vi "MSScript_Format_UpdAuxArbPulses.vi"(9 "ValueArray":string[](array[string]), 10 "TagArray":string[](array[string]), 11 "MSScript.lvclass":refnum<class "MSScript.lvclass">) -> (0 "ValueErrorArray":bool[](array[boolean]), 1 "TagErrorArray":bool[](array[boolean]), 2 "ParamErrorArray":bool[](array[boolean]), 3 "Data":variant, 4 "#ofParamError":bool)   [LabVIEW 2018, in "MSScript.lvclass"]
uses:
  MSScript.lvclass
  Ctl/MSEditorParam updAuxArbPulses.ctl
  MSScript_Transform_EXTArray.vi
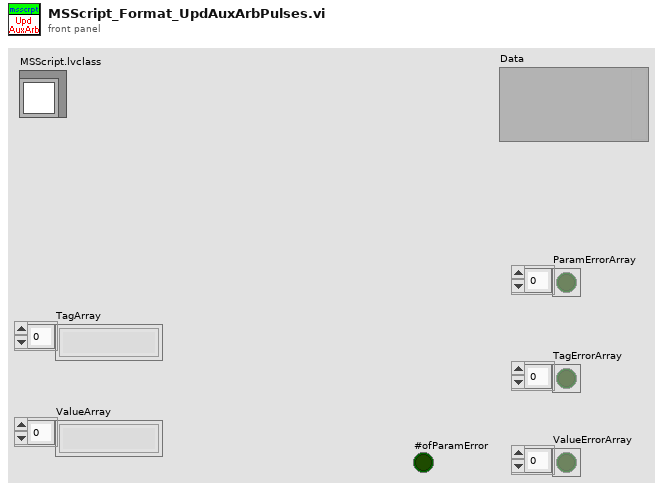
[diagram p1: front panel]
types:
  T1 = typedef "MSEditorParam updAuxArbPulses.ctl" = cluster{"cycleIni":ext[], "cycleEnd":ext[], "pulseInt":ext[]}
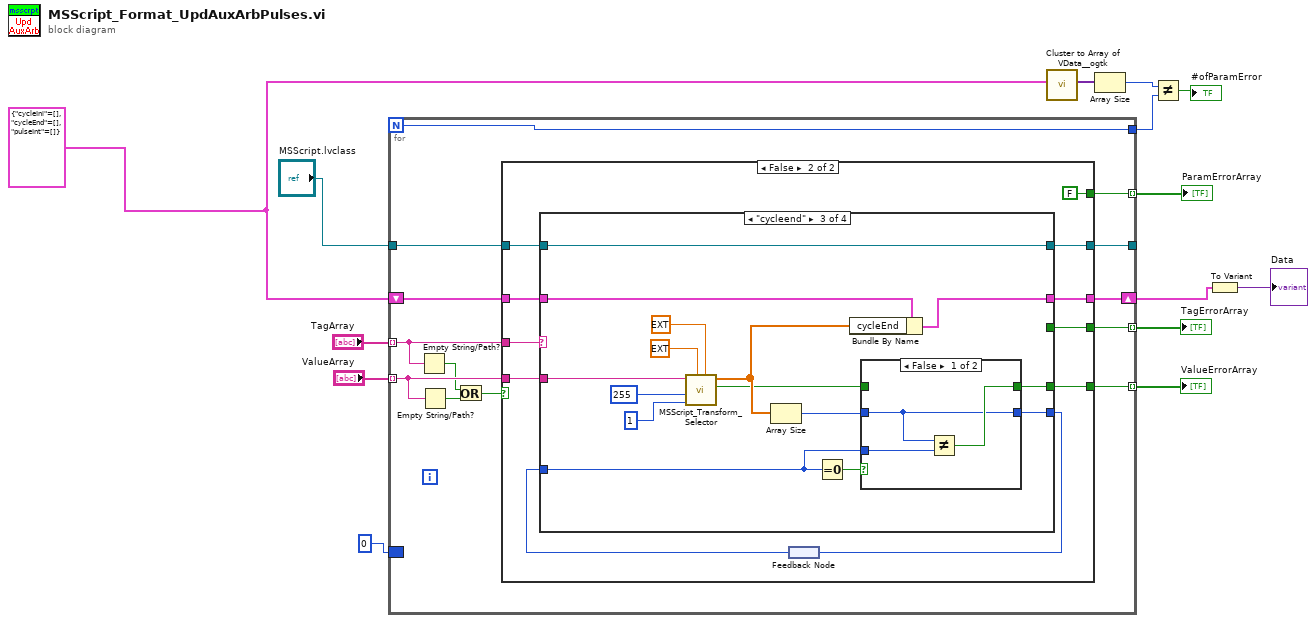
[diagram p0: block diagram]
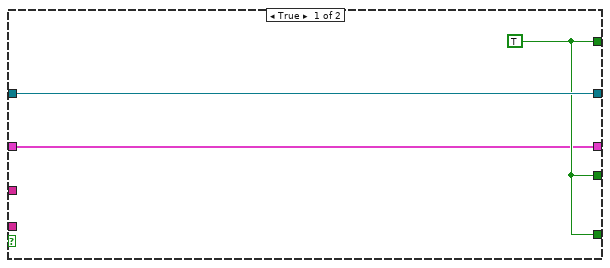
[diagram p2: hidden frame]
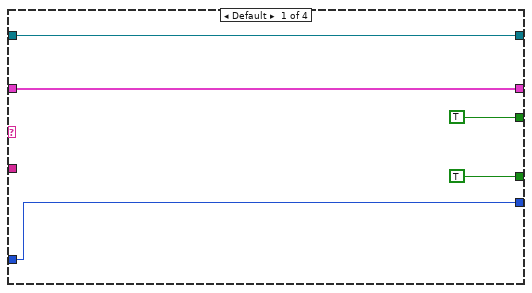
[diagram p3: hidden frame]
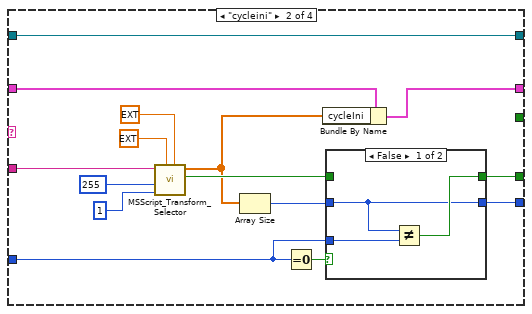
[diagram p4: hidden frame]
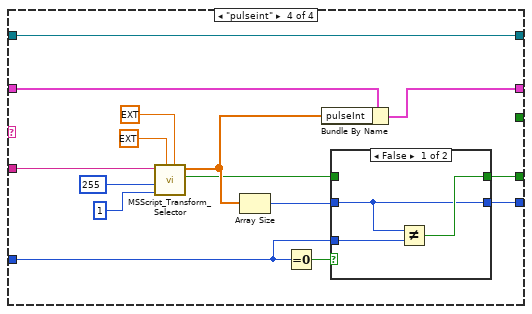
[diagram p7: hidden frame]
diagram:
  w1 = T1 {"cycleIni"=[], "cycleEnd"=[], "pulseInt"=[]} ("Param")
  n1 = for {
    N -> [w15]
    tunnel: "TagArray" -> [w24] mode=indexing
    tunnel: "ValueArray" -> [w23] mode=indexing
    tunnel: [w16] -> w12 mode=indexing
    tunnel: "MSScript.lvclass" -> [w27]
    tunnel: [w26] -> w13 mode=indexing
    tunnel: [w25] -> _
    tunnel: [w19] -> w14 mode=indexing
    shift-right: [w17] -> w3
    shift-left: w1 -> [w18]
    tunnel: [w15] -> w5
    border: 0 -> [_]
    n2 = Empty String/Path?(string/path=w24) -> (empty?=w21:bool)
    n3 = Empty String/Path?(string/path=w23) -> (empty?=w22:bool)
    n4 = Or(x=w21, y=w22) -> (x .or. y?=w20:bool)
    n5 = case shown="False" w20 {
      tunnel: w27 -> [w30 w40]
      tunnel: [w29 w36] -> w26
      tunnel: [w30 w33] -> w25
      tunnel: w24 -> [_ w38]
      tunnel: w23 -> [_ w37]
      tunnel: [w29 FALSE] -> w19
      tunnel: w18 -> [w28 w39]
      tunnel: [w28 w34] -> w17
      tunnel: [w29 w35] -> w16
      frame True {
        w29 = TRUE
      }
      frame False {
        n6 = feedback #1() -> (w31:i32)
        n7 = case shown="\"cycleend\"" w38 {
          tunnel: [TRUE _ _ _] -> w35
          tunnel: w40 -> [w44 w60 w80 w100]
          tunnel: w37 -> [_ w61 w81 w101]
          tunnel: [TRUE ("Value Error?") w53 w68 w87] -> w36
          tunnel: [w44 w60 w80 w100] -> w33
          tunnel: w39 -> [w43 w48 w74 w94]
          tunnel: [w43 w59 w79 w99] -> w34
          tunnel: [w42 w50 w67 w88] -> w32
          tunnel: w31 -> [w42 w49 w72 w90]
          frame Default {
          }
          frame "cycleini" {
            n8 = call-poly "MSScript_Transform_Selector.vi"("upper limit (Inf)"=ext 1.0 ("upper limit"), "lower limit (-Inf)"=ext 0.0 ("lower limit"), "MinSize"=u8 1, "MaxSize"=u8 255, "check_str"=w61) -> ("Value Error?"=w54:bool, "Value Output"=w47:ext[])  [unwired: 4 in, 1 out]
            n9 = Array Size(array=w47) -> (size(s)=w51:i32)
            n10 = Equal To 0?(x=w49) -> (x = 0?=w52:bool)
            n11 = Bundle By Name(cluster=w48, "cycleIni"=w47) -> (w59:T1)
            n12 = case shown="False" w52 {
              tunnel: w51 -> [w62 w65]
              tunnel: [w64 w66] -> w53
              tunnel: w54 -> [_ w66]
              tunnel: [w62 w65] -> w50
              tunnel: w49 -> [w63 _]
              frame False {
                n13 = Not Equal?(x=w62, y=w63) -> (x != y?=w64:bool)
              }
              frame True {
              }
            }
          }
          frame "cycleend" {
            n14 = call-poly "MSScript_Transform_Selector.vi"("upper limit (Inf)"=ext 1.0 ("upper limit"), "lower limit (-Inf)"=ext 0.0 ("lower limit"), "MinSize"=u8 1, "MaxSize"=u8 255, "check_str"=w81) -> ("Value Error?"=w69:bool, "Value Output"=w73:ext[])  [unwired: 4 in, 1 out]
            n15 = Array Size(array=w73) -> (size(s)=w70:i32)
            n16 = Equal To 0?(x=w72) -> (x = 0?=w71:bool)
            n17 = Bundle By Name(cluster=w74, "cycleEnd"=w73) -> (w79:T1)
            n18 = case shown="False" w71 {
              tunnel: w70 -> [w82 w85]
              tunnel: [w84 w86] -> w68
              tunnel: w69 -> [_ w86]
              tunnel: [w82 w85] -> w67
              tunnel: w72 -> [w83 _]
              frame False {
                n19 = Not Equal?(x=w82, y=w83) -> (x != y?=w84:bool)
              }
              frame True {
              }
            }
          }
          frame "pulseint" {
            n20 = call-poly "MSScript_Transform_Selector.vi"("upper limit (Inf)"=ext 1.0 ("upper limit"), "lower limit (-Inf)"=ext -1.0 ("lower limit"), "MinSize"=u8 1, "MaxSize"=u8 255, "check_str"=w101) -> ("Value Error?"=w92:bool, "Value Output"=w93:ext[])  [unwired: 4 in, 1 out]
            n21 = Array Size(array=w93) -> (size(s)=w91:i32)
            n22 = Equal To 0?(x=w90) -> (x = 0?=w89:bool)
            n23 = Bundle By Name(cluster=w94, "pulseInt"=w93) -> (w99:T1)
            n24 = case shown="False" w89 {
              tunnel: w91 -> [w102 w105]
              tunnel: [w104 w106] -> w87
              tunnel: w92 -> [_ w106]
              tunnel: [w102 w105] -> w88
              tunnel: w90 -> [w103 _]
              frame False {
                n25 = Not Equal?(x=w102, y=w103) -> (x != y?=w104:bool)
              }
              frame True {
              }
            }
          }
        }
        n26 = feedback-in #1(w32) -> ()
      }
    }
  }
  "TagErrorArray" <- w12
  "ValueErrorArray" <- w13
  "ParamErrorArray" <- w14
  n27 = call <userlib>:"Cluster to Array of VData__ogtk.vi"("Cluster"=w1) -> ("Array of VData"=w8:variant[])  [unwired: 9 in, 1 out]
  n28 = Array Size(array=w8) -> (size(s)=w7:i32)
  n29 = Not Equal?(x=w7, y=w5) -> (x != y?=→"#ofParamError":bool)
  n30 = To Variant(anything=w3) -> (Variant=→"Data":variant)
